vi "Write SubPanel Ref.vi"(8 "error in (no error)":errorcluster, 10 "SubPanel Ref":refnum<vi>, 11 "Subpanel Inserter in":refnum<class "Subpanel Inserter.lvclass">) -> (0 "error out":errorcluster, 3 "Subpanel Inserter out":refnum<class "Subpanel Inserter.lvclass">)   [LabVIEW 2014, in "Subpanel Insertion.lvlib" / "Subpanel Inserter.lvclass"]
uses:
  Subpanel Inserter.lvclass
  Subpanel Inserter.lvclass/Subpanel Inserter.ctl
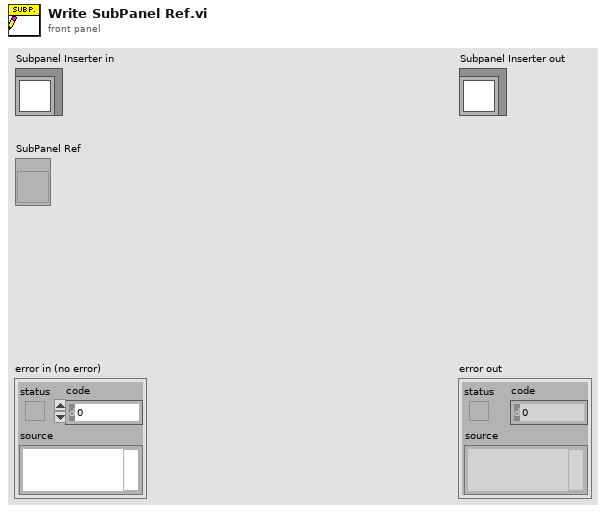
[diagram p1: front panel]
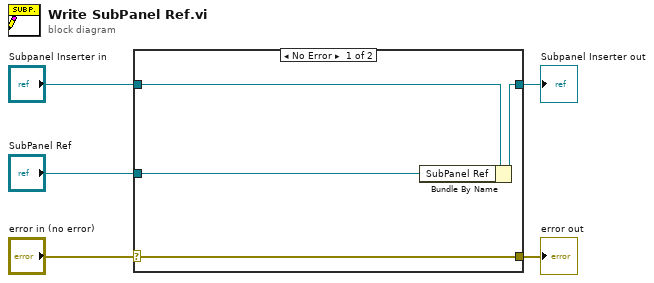
[diagram p0: block diagram]
diagram:
  n1 = case shown="No Error" "error in (no error)" {
    selector: "error in (no error)" -> [w9 w10]
    tunnel: [w9 w10] -> w4
    tunnel: [w7 w11] -> w2
    tunnel: "Subpanel Inserter in" -> [w8 w11]
    tunnel: "SubPanel Ref" -> [w6 _]
    frame No Error {
      n2 = Bundle By Name(cluster=w8, "SubPanel Ref"=w6) -> (w7:refnum<class "Subpanel Inserter.lvclass">)
    }
    frame Error {
    }
  }
  "error out" <- w4
  "Subpanel Inserter out" <- w2
